vi "cmc_acquisition_2.vi"() -> ()   [LabVIEW 2010]
doc: "I. Description:\nThis example demonstrates how to continuously acquire data (waveform) using software timing (rate is governed by while loop iteration interval).\n\nII. Instructions for Running:\n1. Select the physical channel to correspond to where your signal is input on the DAQ device.\n2. Enter the minimum and maximum voltage ranges.\nNote: For better accuracy try to match the input range to the expected voltage level of the measured signal.\n\nIII. Block Diagram Steps:\n1. Create an analog input voltage channel.\n2. Call the Start VI to start the task.\n3. Read the waveform data in a loop until the user hits the stop\nbutton or an error occurs.\n4. Call the Clear Task VI to clear the Task.\n5. Use the popup dialog box to display an error if any.\n\nIV. I/O Connections Overview:\nMake sure your signal input terminal matches the Physical Channel I/O control."
uses:
  <vilib>/Utility/error.llb/DialogType.ctl
  <vilib>/DAQmx/read.llb/DAQmx Read (Analog 1D DBL NChan 1Samp).vi
  <vilib>/DAQmx/create/channels.llb/DAQmx Create Channel (AI-Voltage-Basic).vi
  <vilib>/daqmx/miscellaneous.llb/DAQmx Fill In Error Info.vi
panel:
  in  "units":i32(ring)=10348 items=["Volts"=10348, "SML-10 lbf"=10065]
  in  "Load Limit":dbl
  in  "Scale":tag
  in  "Write to File":bool
  in  "Software Loop Time (ms)":u32=250
  in  "Physical Channel":tag="Dev1/ai0"
  in  "Minimum Value":dbl=-10.0 format="%0.2f"
  in  "Maximum Value":dbl=10.0 format="%0.2f"
  in  "stop":bool
  out "Measurement":dbl[](graph)
  # "For instructions, select Help>>Show Context Help"
  # "Timing Parameters"
  # "Channel Parameters"
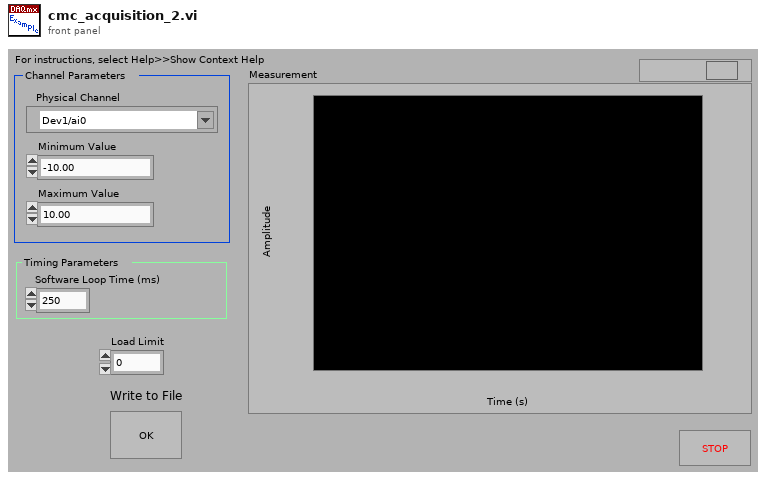
[diagram p1: front panel]
types:
  T1 = enum16{"open", "replace", "create", "open or create", "replace or create", "replace or create with confirmation"}
  T2 = typedef "DialogType.ctl" = u16
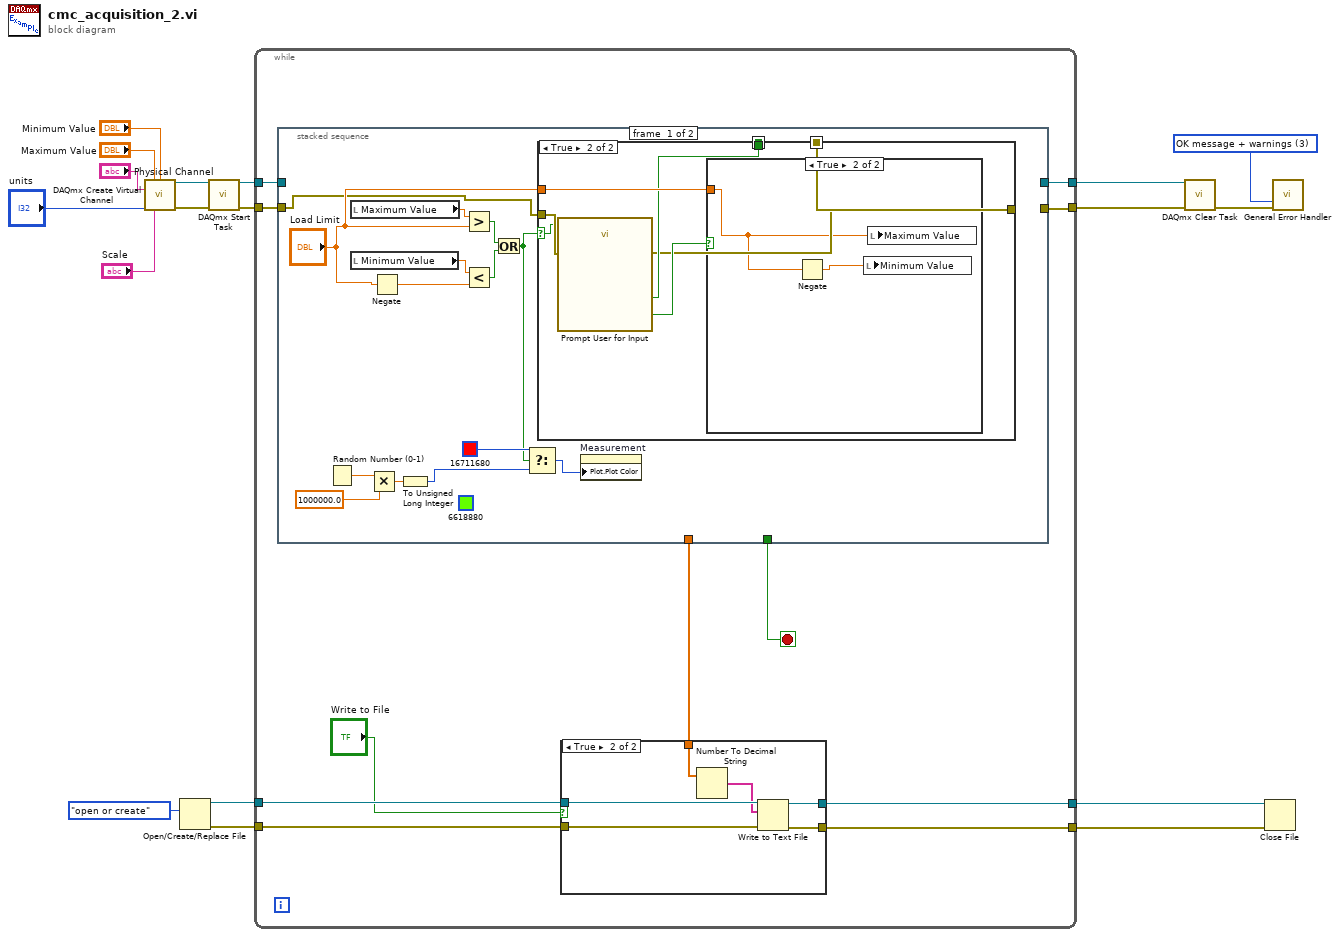
[diagram p0: block diagram]
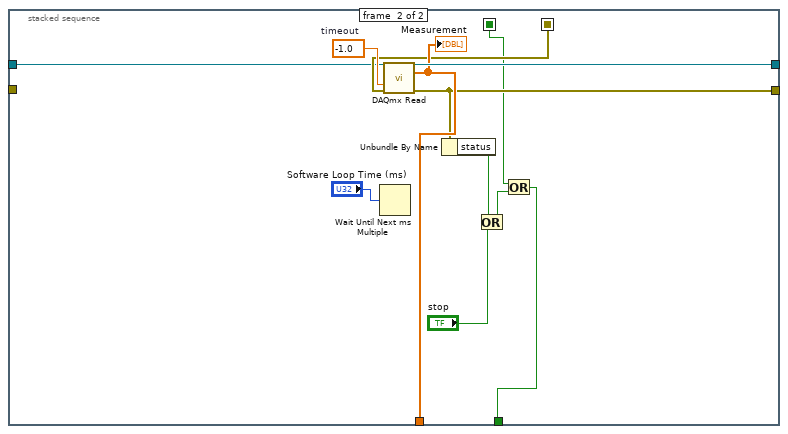
[diagram p4: hidden frame]
diagram:
  w8 = T2 3 items=["no dialog", "OK message", "continue or stop message", "OK message + warnings", "continue/stop + warnings"] ("type of dialog (OK msg:1)")
  n1 = call-poly <vilib>:"DAQmx Create Virtual Channel.vi"("maximum value"="Maximum Value", "minimum value"="Minimum Value", "physical channels"="Physical Channel", "units"="units", "custom scale name"="Scale") -> ("task out"=w10:refnum<k21>, "error out"=w9:errorcluster)  [unwired: 9 in]
  n2 = Open/Create/Replace File(operation (0:open)=T1."open or create") -> (refnum out=w6:refnum<file>, error out=w5:errorcluster)  [unwired: 5 in, 1 out]
  n3 = call <vilib>:"DAQmx Start Task.vi"("task/channels in"=w10, "error in"=w9) -> ("task out"=w13:refnum<k21>, "error out"=w16:errorcluster)  [unwired: 12 in]
  n4 = while {
    tunnel: w16 -> [w29]
    tunnel: [w21] -> w15
    tunnel: w13 -> [w19]
    tunnel: [w27] -> w12
    tunnel: w6 -> [w26]
    tunnel: w5 -> [w25]
    tunnel: [w24] -> w4
    tunnel: [w23] -> w3
    stop <- w28 stop-if-true
    n5 = stacked-sequence {
      seq-local: [w36 _] -> [_ w57]
      seq-local: [w39 _] -> [_ w61]
      tunnel: w29 -> [w38 _]
      tunnel: [_ w59] -> w28
      tunnel: [_ w65] -> w27
      tunnel: [_ w63] -> w22
      tunnel: [_ w58] -> w21
      tunnel: w19 -> [_ w56]
      frame #0 {
        (unwired) u32 6618880
        n6 = Random Number (0-1)() -> (number: 0 to 1=w34:dbl)
        n7 = local read "Maximum Value"() -> (w43:dbl)
        n8 = local read "Minimum Value"() -> (w42:dbl)
        n9 = Multiply(x=w34, y=1000000.0) -> (x*y=w32:dbl)
        n10 = Negate(x="Load Limit") -> (-x=w41:dbl)
        n11 = To Unsigned Long Integer(number=w32) -> (unsigned 32bit integer=w30:u32)
        n12 = Greater?(x=w43, y="Load Limit") -> (0:w44:bool)
        n13 = Less?(x=w42, y=w41) -> (x < y?=w45:bool)
        n14 = Or(x=w44, y=w45) -> (x .or. y?=w35:bool)
        n15 = Select(t=u32 16711680, s=w35, f=w30) -> (s? t:f=w31:u32)
        n16 = case shown="True" w35 {
          selector: w35 -> [w46 w51]
          tunnel: "Load Limit" -> [_ w53]
          tunnel: [w47 w48] -> w39
          tunnel: w38 -> [w47 w52]
          tunnel: [w46 w50] -> w36
          frame False {
          }
          frame True {
            n17 = call "Prompt User for Input"("Enable"=w51, "error in (no error)"=w52) -> ("Yes"=w49:bool, "OK"=w50:bool, "error out"=w48:errorcluster)  [unwired: 15 in]
            n18 = case shown="True" w49 {
              tunnel: w53 -> [_ w54]
              frame False {
              }
              frame True {
                n19 = Negate(x=w54) -> (-x=w55:dbl)
                n20 = local write "Minimum Value"(w55) -> ()
                n21 = local write "Maximum Value"(w54) -> ()
              }
            }
          }
        }
        n22 = property on="Measurement" class="WFChart (strict)"("Plot.Plot Color"=w31) -> ()  [unwired: 2 in, 2 out]
      }
      frame #1 {
        w62 = -1.0  # timeout
        n23 = Wait Until Next ms Multiple(millisecond multiple="Software Loop Time (ms)") -> ()  [unwired: 1 out]
        n24 = call-poly <vilib>:"DAQmx Read.vi"("task/channels in"=w56, "timeout"=w62, "error in"=w61) -> ("task out"=w65:refnum<k21>, "data"=w63:dbl[], "error out"=w58:errorcluster)  [unwired: 10 in]
        "Measurement" <- w63
        n25 = Unbundle By Name(w58) -> ("status"=w66:bool)
        n26 = Or(x=w66, y="stop") -> (x .or. y?=w60:bool)
        n27 = Or(x=w57, y=w60) -> (x .or. y?=w59:bool)
      }
    }
    n28 = case shown="True" "Write to File" {
      tunnel: w26 -> [w69 w75]
      tunnel: w25 -> [w68 w74]
      tunnel: [w69 w73] -> w24
      tunnel: [w68 w72] -> w23
      tunnel: w22 -> [_ w71]
      frame False {
      }
      frame True {
        n29 = Number To Decimal String(number=w71) -> (decimal integer string=w70:string[])  [unwired: 1 in]
        n30 = Write to Text File(file (use dialog)=w75, text=w70, error in=w74) -> (refnum out=w73:refnum<file>, error out=w72:errorcluster)  [unwired: 1 in, 1 out]
      }
    }
  }
  n31 = call <vilib>:"DAQmx Clear Task.vi"("task in"=w12, "error in"=w15) -> ("error out"=w14:errorcluster)  [unwired: 13 in]
  n32 = Close File(refnum=w4, error in=w3) -> ()  [unwired: 2 out]
  n33 = call <vilib>:"General Error Handler.vi"("type of dialog (OK msg:1)"=w8, "error in (no error)"=w14) -> ()  [unwired: 9 in, 5 out]
